vi "Loop_ACT_Left_Motor.vi"() -> ()   [LabVIEW 2017, in "Claw.lvlib"]
uses:
  Claw.lvlib
  TypeDef/CLUSTER_Two Motor Input.ctl
  Globals/Global_Device_IDs.vi
  <vilib>/Rock Robotics/WPI/RobotDrive/WPI_RobotDriveOpen2MotorWithVictorSP.vi
  _SHARE ALL/Global Share All/Global_STOP.vi
  Global_SM Write_Data Out.vi
  Global_ACT Write_Data Out.vi
panel:
  out "Claw Output":T1
  out "Cycle Time (S)":dbl format="%.3g"
  in  "Target Time(ms)":u32=50
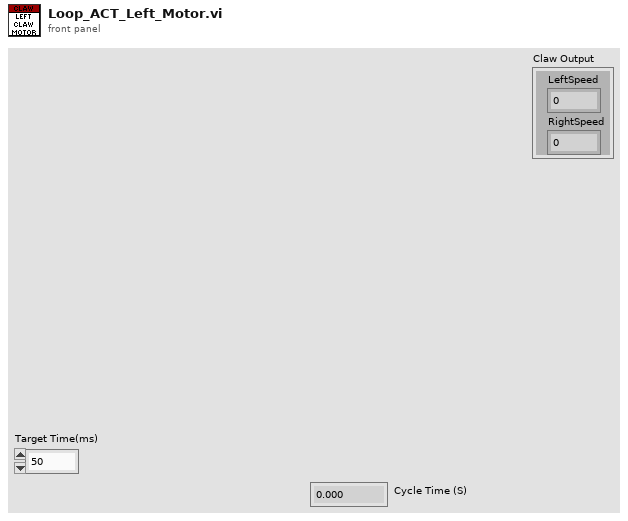
[diagram p1: front panel]
types:
  T1 = typedef "CLUSTER_Two Motor Input.ctl" = cluster{"LeftSpeed":dbl, "RightSpeed":dbl}
  T2 = typedef "CLUSTER_Claw_Setup.ctl" = cluster{"Left Motor Setup":T3, "Right Motor Setup":T3}
  T3 = typedef "CLUSTER_PWM Motor Setup.ctl" = cluster{"Motor PWM":T4, "Invert Motor":bool}
  T4 = typedef "FPGA_DIOPWMChannel.ctl" = enum8{"PWM 0", "PWM 1", "PWM 2", "PWM 3", "PWM 4", "PWM 5", "PWM 6", "PWM 7", "PWM 8", "PWM 9", "PWM MXP 0", "PWM MXP 1", "PWM MXP 2", "PWM MXP 3", "PWM MXP 4", "PWM MXP 5", "PWM MXP 6", "PWM MXP 7", "PWM MXP 8", "PWM MXP 9", "Invalid"}
  T5 = typedef "WPI_RobotDriveDevRef.ctl" = cluster{"DevStatus":errorcluster, "Motors[]":T6[], "Square Inputs":bool, "Max Output":dbl}
  T6 = typedef "WPI_MotorControlDeviceRef.ctl" = cluster{"DeviceStatus":errorcluster, "Type":T7, "PWM":cluster{"PWM Channel":T4, "DeadBand":T8}, "CAN":cluster{"Device Number":u8, "SetOutput VI Ref":variant, "GetOutput VI Ref":variant, "Enable VI Ref":variant, "Disable VI Ref":variant, "Data":variant}, "Invert":bool, "DIO PWM":cluster{"PWM \"Enable\" Channel":T4, "DIOChannel":T9, "PWM Rate":dbl}}
  T7 = typedef "WPI_MotorControlType.ctl" = enum16{"PWM", "CAN", "DIO PWM"}
  T8 = typedef "WPI_PWMDeadband.ctl" = cluster{"Name":string, "maxPositivePwm":i32, "minPositivePwm":i32, "centerPwm":i32, "maxNegativePwm":i32, "minNegativePwm":i32, "angularRange":u16}
  T9 = typedef "FPGA_DIOChannel.ctl" = enum8{"DIO 0", "DIO 1", "DIO 2", "DIO 3", "DIO 4", "DIO 5", "DIO 6", "DIO 7", "DIO 8", "DIO 9", "DIO MXP 0", "DIO MXP 1", "DIO MXP 2", "DIO MXP 3", "DIO MXP 4", "DIO MXP 5", "DIO MXP 6", "DIO MXP 7", "DIO MXP 8", "DIO MXP 9", "DIO MXP 10", "DIO MXP 11", "DIO MXP 12", "DIO MXP 13", "DIO MXP 14", "DIO MXP 15", "SPI Port CS1", "SPI Port CS2", "SPI Port CS3", "SPI Port MISO", "SPI Port MOSI", "Invalid"}
  T10 = cluster{"RobotDriveDevRef":T5, "Claw Output":T1, "Claw Input":T1, "Target Time(ms)":u32, "Current Time":timestamp, "Previous Time":timestamp, "Cycle Time (S)":dbl}
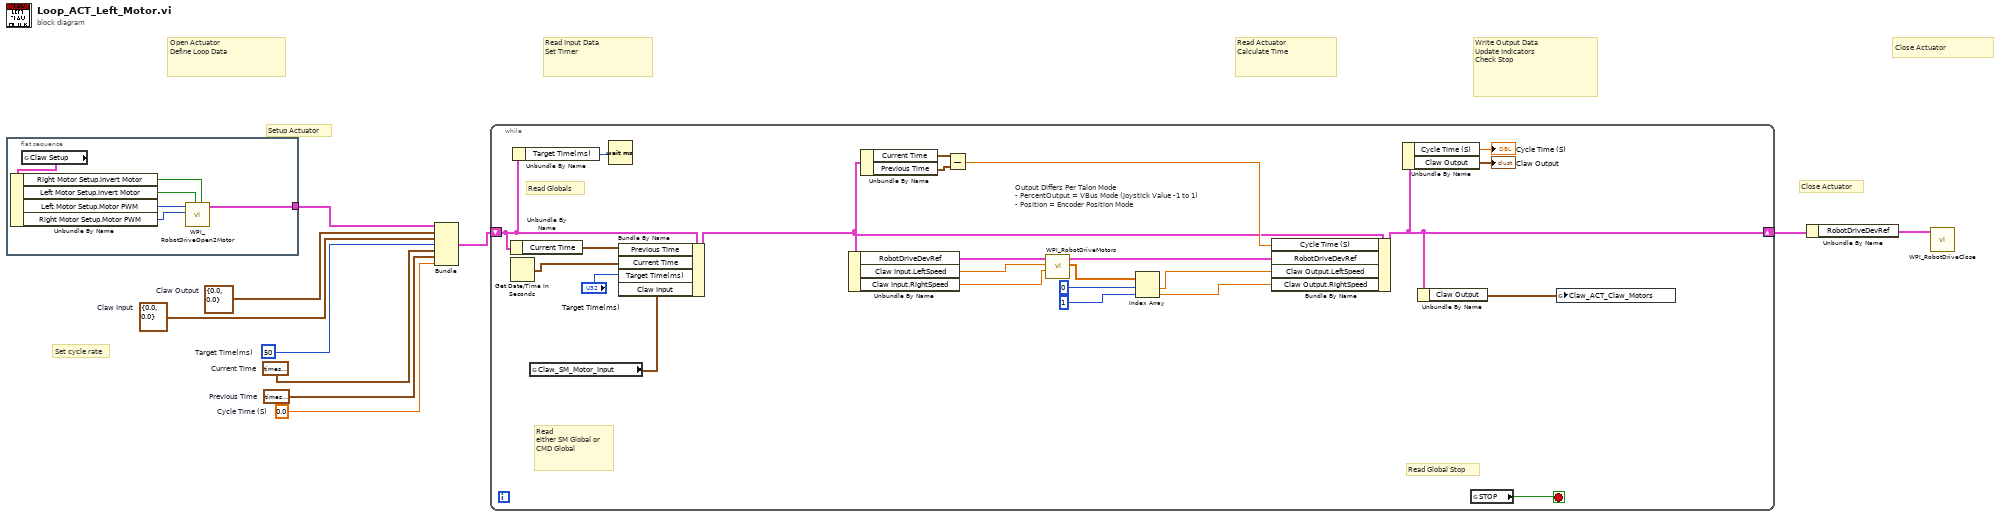
[diagram p0: block diagram]
diagram:
  w2 = T1 {"LeftSpeed"=0.0, "RightSpeed"=0.0}  # Claw Output
  w3 = T1 {"LeftSpeed"=0.0, "RightSpeed"=0.0}  # Claw Input
  w5 = 0.0  # Cycle Time (S)
  w10 = timestamp(0 s since 1904-01-01)  # Previous Time
  w9 = timestamp(0 s since 1904-01-01)  # Current Time
  w8 = u32 50  # Target Time(ms)
  # "Close Actuator"
  # "Write Output Data\nUpdate Indicators\nCheck Stop"
  # "Read Actuator\nCalculate Time"
  # "Read Input Data\nSet Timer"
  # "Open Actuator\nDefine Loop Data"
  # "Set cycle rate"
  # "Close Actuator"
  # "Setup Actuator"
  n1 = flat-sequence {
    tunnel: [w15] -> w4
    frame #0 {
      n2 = global read "Global_Device_IDs.vi" "Claw Setup"() -> (w16:T2)
      n3 = Unbundle By Name(w16) -> ("Right Motor Setup.Invert Motor"=w14:bool, "Left Motor Setup.Invert Motor"=w13:bool, "Left Motor Setup.Motor PWM"=w12:T4, "Right Motor Setup.Motor PWM"=w11:T4)
      n4 = call-poly <vilib>:"WPI_RobotDriveOpen2Motor.vi"("Right Motor Inverted"=w14, "Left Motor Inverted"=w13, "Right Motor"=w11, "Left Motor"=w12) -> ("RobotDriveDevRef"=w15:T5)  [unwired: 6 in, 1 out]
    }
  }
  n5 = Bundle("RobotDriveDevRef"=w4, "Claw Output"=w2, "Claw Input"=w3, "Target Time(ms)"=w8, "Current Time"=w9, "Previous Time"=w10, "Cycle Time (S)"=w5) -> (w7:T10)  [unwired: 1 in]
  n6 = while {
    shift-right: [w32] -> w6
    shift-left: w7 -> [w34]
    stop <- w40 stop-if-true
    # "Output Differs Per Talon Mode\n- PercentOutput = VBus Mode (Joystick Value -1 to 1)\n- Position = Encoder Position Mode"
    # "Read\neither SM Global or CMD Global"
    # "Read Globals"
    # "Read Global Stop"
    n7 = Unbundle By Name(w34) -> ("Current Time"=w38:timestamp)
    n8 = Get Date/Time In Seconds() -> (seconds since 1Jan1904=w39:timestamp)
    n9 = Unbundle By Name(w34) -> ("Target Time(ms)"=w33:u32)
    n10 = global read "Global_SM Write_Data Out.vi" "Claw_SM_Motor_Input"() -> (w28:T1)
    n11 = Wait (ms)(milliseconds to wait=w33) -> ()  [unwired: 1 out]
    n12 = Bundle By Name(cluster=w34, "Previous Time"=w38, "Current Time"=w39, "Target Time(ms)"="Target Time(ms)", "Claw Input"=w28) -> (w29:T10)
    n13 = Unbundle By Name(w29) -> ("RobotDriveDevRef"=w26:T5, "Claw Input.LeftSpeed"=w25:dbl, "Claw Input.RightSpeed"=w24:dbl)
    n14 = Unbundle By Name(w29) -> ("Current Time"=w37:timestamp, "Previous Time"=w36:timestamp)
    n15 = Subtract(x=w37, y=w36) -> (x-y=w30:dbl)
    n16 = call <vilib>:"WPI_RobotDriveMotors.vi"("RightSpeed"=w24, "LeftSpeed"=w25, "RobotDriveDevRef"=w26) -> ("Motor Values"=w23:dbl[], "RobotDriveDevRef"=w18:T5)  [unwired: 6 in, 1 out]
    n17 = Index Array(array=w23, index #1=0 ("index"), index #2=1 ("index")) -> (element #1=w20:dbl, element #2=w19:dbl)
    n18 = Bundle By Name(cluster=w29, "Cycle Time (S)"=w30, "RobotDriveDevRef"=w18, "Claw Output.LeftSpeed"=w20, "Claw Output.RightSpeed"=w19) -> (w32:T10)
    n19 = Unbundle By Name(w32) -> ("Cycle Time (S)"=→"Cycle Time (S)":dbl, "Claw Output"=→"Claw Output":T1)
    n20 = Unbundle By Name(w32) -> ("Claw Output"=w27:T1)
    n21 = global read "Global_STOP.vi" "STOP"() -> (w40:bool)
    n22 = global write "Global_ACT Write_Data Out.vi" "Claw_ACT_Claw_Motors"(w27) -> ()
  }
  n23 = Unbundle By Name(w6) -> ("RobotDriveDevRef"=w1:T5)
  n24 = call <vilib>:"WPI_RobotDriveClose.vi"("RobotDriveDevRef"=w1) -> ()  [unwired: 10 in, 1 out]
